vi "Write Connection.vi"(8 "error in (no error)":errorcluster, 10 "Connection":refnum<k5>, 11 "TrialBasedExperiment in":refnum<class "MatlabExperiment.lvclass">) -> (0 "error out":errorcluster, 3 "TrialBasedExperiment out":refnum<class "MatlabExperiment.lvclass">)   [LabVIEW 2010, in "MatlabExperiment.lvclass"]
uses:
  MatlabExperiment.lvclass
  MatlabExperiment.lvclass/MatlabExperiment.ctl
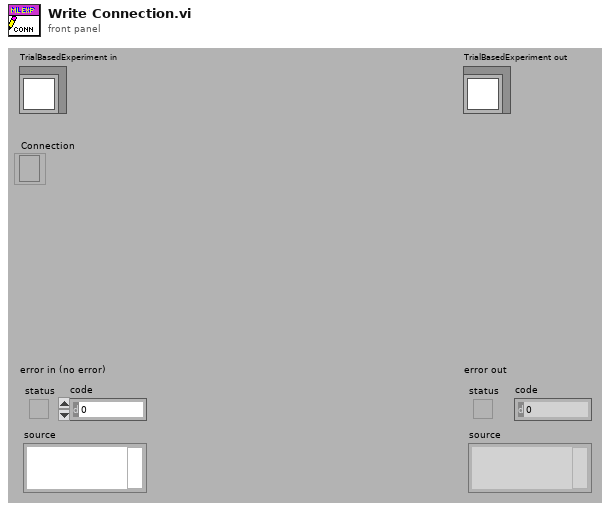
[diagram p1: front panel]
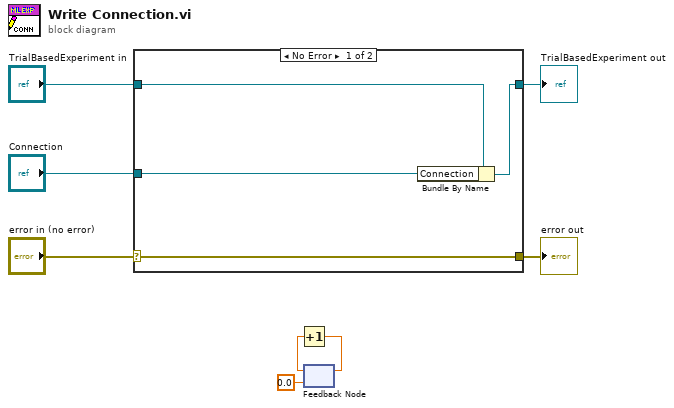
[diagram p0: block diagram]
diagram:
  n1 = case shown="No Error" "error in (no error)" {
    selector: "error in (no error)" -> [w12 w13]
    tunnel: [w12 w13] -> w7
    tunnel: [w10 w14] -> w5
    tunnel: "TrialBasedExperiment in" -> [w11 w14]
    tunnel: "Connection" -> [w9 _]
    frame No Error {
      n2 = Bundle By Name(cluster=w11, "Connection"=w9) -> (w10:refnum<class "MatlabExperiment.lvclass">)
    }
    frame Error {
    }
  }
  "error out" <- w7
  "TrialBasedExperiment out" <- w5
  n3 = feedback #1(0.0) -> (w3:dbl)
  n4 = Increment(x=w3) -> (x+1=w2:dbl)
  n5 = feedback-in #1(w2) -> ()
